vi "Tell Child.vi"(4 "Priority":bool, 6 "UID":string, 7 "Actor in":refnum<class "Actor.lvclass">, 10 "Msg":refnum<class "Msg.lvclass">) -> (0 "Error out":errorcluster)   [LabVIEW 2025, in "jettl.lvlib"]
uses:
  jettl.lvlib
  Relation.ctl
  Teller/Teller.lvlib
  Actor/Actor.lvclass
  Transport/Transport/Transport.lvclass
  Msg/Msg.lvclass
  Attributes/Attributes/Attributes.lvclass
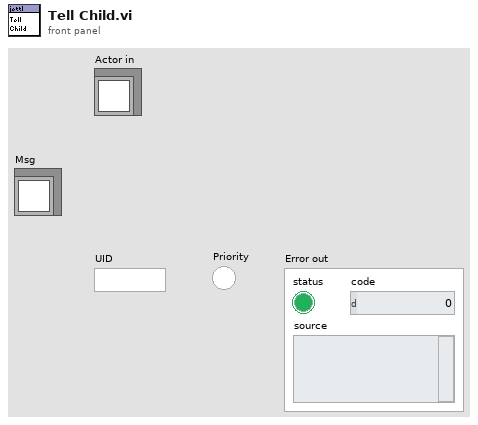
[diagram p1: front panel]
types:
  T1 = typedef "jettl.lvlib/Relation.ctl" = enum16{"Self", "Parent", "Child"}
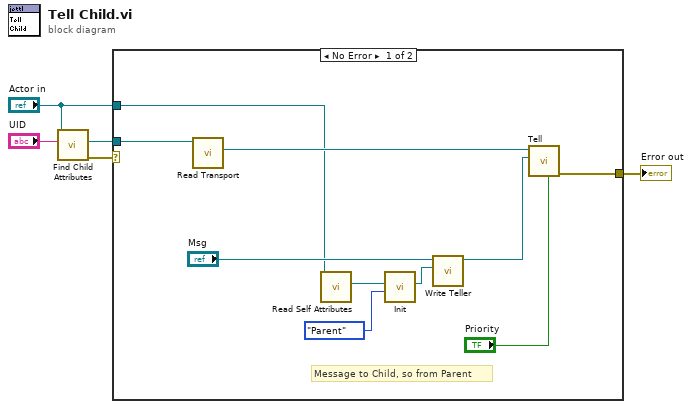
[diagram p0: block diagram]
diagram:
  n1 = call-dynamic "Find Child Attributes.vi"("UID"="UID", "Actor in"="Actor in") -> ("Error out"=w3:errorcluster, "Child Attributes"=w2:refnum<class "Attributes.lvclass">)  [unwired: 8 in]
  n2 = case shown="No Error" w3 {
    selector: w3 -> [_ w16]
    tunnel: "Actor in" -> [w12 _]
    tunnel: [w15 w16] -> w5
    tunnel: w2 -> [w11 _]
    frame No Error {
      # "Message to Child, so from Parent"
      n3 = call-dynamic "Read Transport.vi"("Attributes in"=w11) -> ("Transport"=w14:refnum<class "Transport.lvclass">)  [unwired: 10 in]
      n4 = call-dynamic "Read Self Attributes.vi"("Actor in"=w12) -> ("Self Attributes"=w8:refnum<class "Attributes.lvclass">)  [unwired: 10 in]
      n5 = call "Init.vi"("Relation"=Relation."Parent", "Self Attributes"=w8) -> ("Teller"=w10:refnum<class "Teller.lvclass">)  [unwired: 9 in]
      n6 = call-dynamic "Write Teller.vi"("Teller"=w10, "Msg in"="Msg") -> ("Msg out"=w7:refnum<class "Msg.lvclass">)  [unwired: 9 in]
      n7 = call-dynamic "Tell.vi"("Priority"="Priority", "Msg"=w7, "Transport in"=w14) -> ("Error out"=w15:errorcluster)  [unwired: 8 in]
    }
    frame Error {
    }
  }
  "Error out" <- w5
